vi "Execute Msg.vi"(7 "Actor in":refnum<class "Actor.lvclass">, 8 "Error in":errorcluster, 11 "Stop Msg in":refnum<class "Stop Msg.lvclass">) -> (0 "Error out":errorcluster, 2 "Msg Output":refnum<class "Msg Output.lvclass">, 5 "Actor out":refnum<class "Actor.lvclass">)   [LabVIEW 2025, in "jettl.lvlib" / "Stop jettl Msg.lvlib" / "Stop Msg.lvlib" / "Stop Msg.lvclass"]
uses:
  Stop Msg.lvclass
  Stop Msg.lvclass/Stop Msg.ctl
  Stop jettl Msg/Stop jettl Msg.lvclass
  Actor/Actor.lvclass
  Msg Output/Msg Output.lvclass
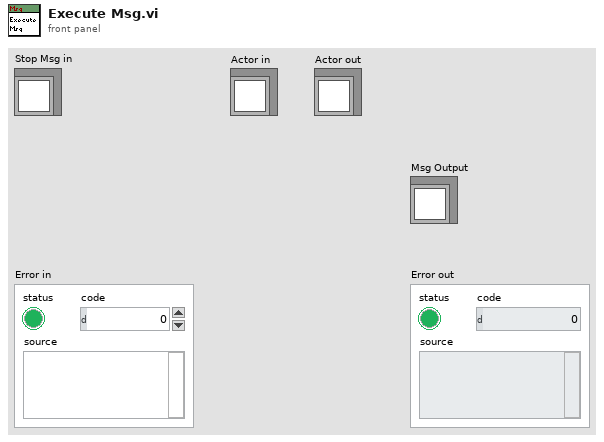
[diagram p1: front panel]
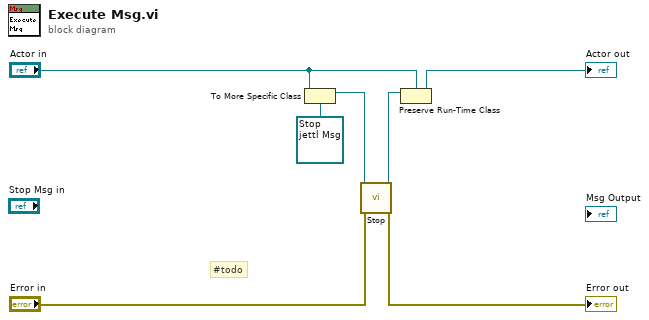
[diagram p0: block diagram]
diagram:
  # "#todo"
  n1 = To More Specific Class(target class=refnum<class "Stop jettl Msg.lvclass"> refnum ("jettl.lvlib:Stop jettl Msg.lvlib:Stop jettl Msg.lvclass"), reference="Actor in") -> (specific class reference=w5:refnum<class "Stop jettl Msg.lvclass">)  [unwired: 1 in, 1 out]
  n2 = call-dynamic "Stop.vi"("Error in"="Error in", "Stop jettl Msg in"=w5) -> ("Error out"=→"Error out":errorcluster, "Stop jettl Msg out"=w4:refnum<class "Stop jettl Msg.lvclass">)  [unwired: 8 in]
  n3 = Preserve Run-Time Class(object in=w4, 2:"Actor in") -> (object out=→"Actor out":refnum<class "Actor.lvclass">)  [unwired: 1 in, 1 out]
